vi "Open Client Connection.vi"(8 "error in (no error)":errorcluster, 9 "Port":u16, 10 "address":string, 11 "RemoteControl.STM in":refnum<class "RemoteControl.STM.lvclass">) -> (0 "error out":errorcluster, 3 "RemoteControl.STM out":refnum<class "RemoteControl.STM.lvclass">)   [LabVIEW 2016, in "RemoteControl.STM.lvclass"]
uses:
  RemoteControl.STM.lvclass
  RemoteControl.STM.lvclass/RemoteControl.STM.ctl
  <vilib>/NI/STM/TCP/Read Meta Data (TCP Ref).vi
  <vilib>/NI/STM/TCP/Read Meta Data (TCP Clst).vi
  <vilib>/NI/STM/NI STM.lvlib
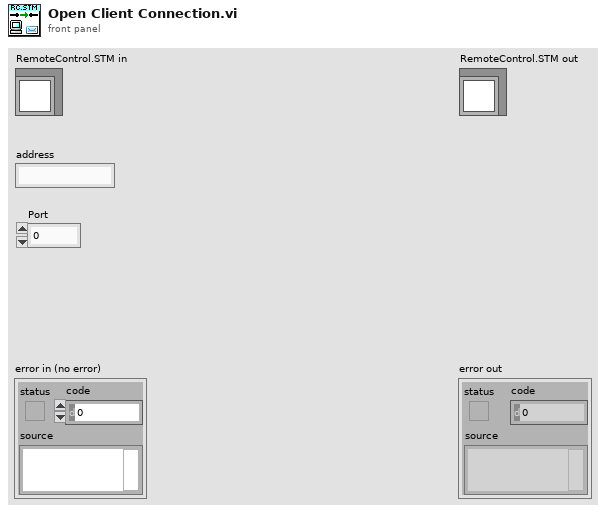
[diagram p1: front panel]
types:
  T1 = typedef "NI STM.lvlib/TCP Connection Info.ctl" = cluster{"connection ID":refnum<k5>, "meta data":T2[]}
  T2 = typedef "NI STM.lvlib/MetaDataElement.ctl" = string
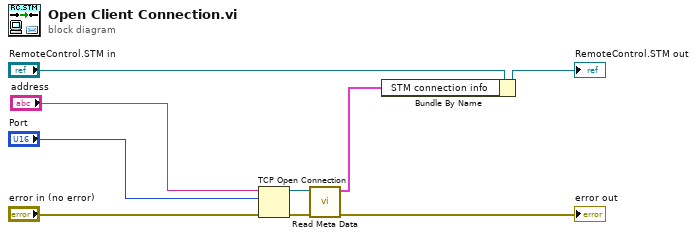
[diagram p0: block diagram]
diagram:
  n1 = TCP Open Connection(address="address", remote port or service name="Port", error in (no error)="error in (no error)") -> (connection ID=w8:refnum<k5>, error out=w9:errorcluster)  [unwired: 2 in]
  n2 = call-poly <vilib>:"Read Meta Data.vi"("error in"=w9, "connection ID"=w8) -> ("error out"=→"error out":errorcluster, "connection info out"=w6:T1)  [unwired: 7 in, 1 out]
  n3 = Bundle By Name(cluster="RemoteControl.STM in", "STM connection info"=w6) -> (→"RemoteControl.STM out":refnum<class "RemoteControl.STM.lvclass">)
